vi "Judge.vi"(1 "Dealer's card":i32[](array[numeric]), 2 "Player's card":i32[](array[numeric])) -> (0 "Output result":i32)   [LabVIEW 2018]
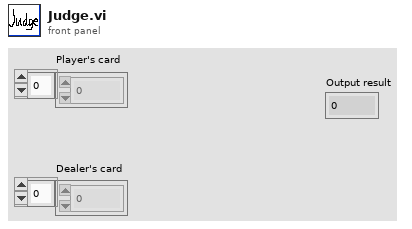
[diagram p1: front panel]
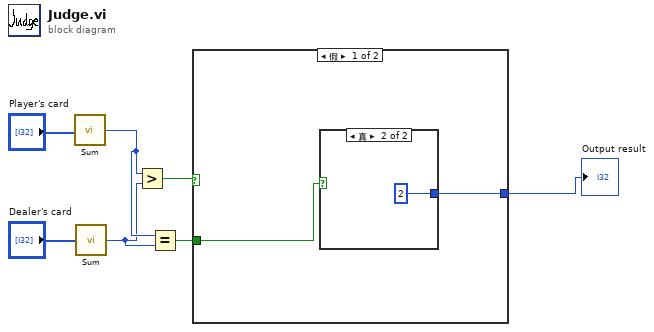
[diagram p0: block diagram]
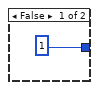
[diagram p2: hidden frame]
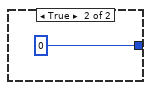
[diagram p3: hidden frame]
diagram:
  n1 = call "Sum.vi"("Array"="Player's card") -> ("Value"=w4:i32)
  n2 = call "Sum.vi"("Array"="Dealer's card") -> ("Value"=w3:i32)
  n3 = Greater?(x=w4, y=w3) -> (0:w5:bool)
  n4 = Equal?(x=w4, y=w3) -> (x = y?=w1:bool)
  n5 = case shown="假" w5 {
    tunnel: [w8 0] -> w2
    tunnel: w1 -> [w9 _]
    frame False {
      n6 = case shown="真" w9 {
        tunnel: [1 2] -> w8
        frame False {
        }
        frame True {
        }
      }
    }
    frame True {
    }
  }
  "Output result" <- w2
